vi "Pre-Install Custom Action.vi"(10 "Variant":variant) -> (0 "error out":errorcluster)   [LabVIEW 2021]
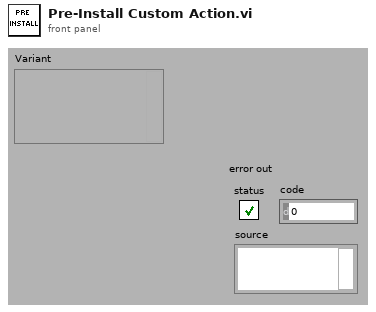
[diagram p1: front panel]
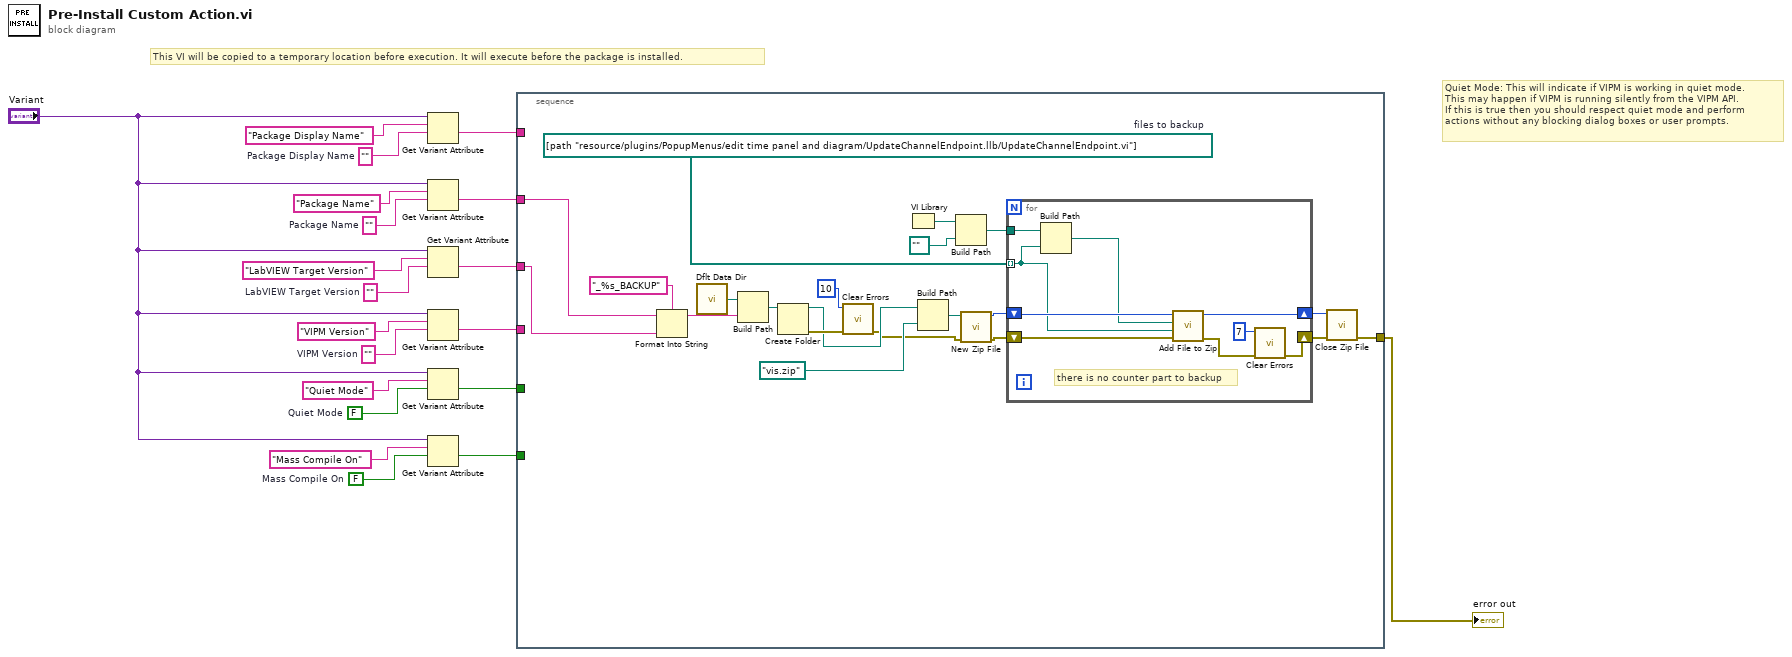
[diagram p0: block diagram]
diagram:
  w2 = FALSE  # Mass Compile On
  w4 = ""  # Package Display Name
  w11 = FALSE  # Quiet Mode
  w14 = ""  # VIPM Version
  w16 = ""  # LabVIEW Target Version
  w18 = ""  # Package Name
  # "Quiet Mode: This will indicate if VIPM is working in quiet mode.\nThis may happen if VIPM is running silently from the VIPM API.\nIf this is true then you should respect quiet mode and perform\nactions without any blocking dialog boxes or user prompts."
  # "This VI will be copied to a temporary location before execution. It will execute before the package is installed."
  n1 = Get Variant Attribute(Variant="Variant", name="Package Display Name", default value (empty Variant)=w4) -> (value=w10:string)  [unwired: 1 in, 3 out]
  n2 = Get Variant Attribute(Variant="Variant", name="Package Name", default value (empty Variant)=w18) -> (value=w9:string)  [unwired: 1 in, 3 out]
  n3 = Get Variant Attribute(Variant="Variant", name="LabVIEW Target Version", default value (empty Variant)=w16) -> (value=w8:string)  [unwired: 1 in, 3 out]
  n4 = Get Variant Attribute(Variant="Variant", name="VIPM Version", default value (empty Variant)=w14) -> (value=w7:string)  [unwired: 1 in, 3 out]
  n5 = Get Variant Attribute(Variant="Variant", name="Quiet Mode", default value (empty Variant)=w11) -> (value=w6:bool)  [unwired: 1 in, 3 out]
  n6 = Get Variant Attribute(Variant="Variant", name="Mass Compile On", default value (empty Variant)=w2) -> (value=w5:bool)  [unwired: 1 in, 3 out]
  n7 = stacked-sequence {
    tunnel: w10 -> [_]
    tunnel: w9 -> [w40]
    tunnel: w8 -> [w39]
    tunnel: w7 -> [_]
    tunnel: w6 -> [_]
    tunnel: w5 -> [_]
    tunnel: [w21] -> w1
    frame #0 {
      w29 = path[] [path "resource/plugins/PopupMenus/edit time panel and diagram/UpdateChannelEndpoint.llb/UpdateChannelEndpoint.vi"]  # files to backup
      n8 = Format Into String(format string="_%s_BACKUP", initial string=w40, w39) -> (resulting string=w27:string)  [unwired: 1 in, 1 out]
      n9 = call <vilib>:"Dflt Data Dir.vi"() -> ("App:Default Data Directory"=w28:path)
      n10 = Build Path(base path=w28, name or relative path=w27) -> (appended path=w26:path)
      n11 = Create Folder(path (use dialog)=w26) -> (created path=w23:path, error out=w25:errorcluster)  [unwired: 2 in, 1 out]
      n12 = call <vilib>:"Clear Errors.vi"("error in (no error)"=w25, "specific error code to clear (0: all)"=10) -> ("error out"=w22:errorcluster)  [unwired: 4 in, 1 out]
      n13 = VI Library() -> (path=w34:path)
      n14 = Build Path(base path=w23, name or relative path=path "vis.zip") -> (appended path=w30:path)
      n15 = Build Path(base path=w34, name or relative path=path "..") -> (appended path=w32:path)
      n16 = call <vilib>:"New Zip File.vi"("error in (no error)"=w22, "target"=w30) -> ("error out"=w37:errorcluster, "zip file out"=w38:i64)  [unwired: 3 in, 1 out]
      n17 = for {
        tunnel: w29 -> [w42] mode=indexing
        shift-right: [w45] -> w36
        shift-left: w37 -> [w47]
        shift-right: [w48] -> w35
        shift-left: w38 -> [w49]
        tunnel: w32 -> [w43]
        # "there is no counter part to backup"
        n18 = Build Path(base path=w43, name or relative path=w42) -> (appended path=w46:path)
        n19 = call <vilib>:"Add File to Zip.vi"("error in (no error)"=w47, "destination path in zip"=w42, "source file path"=w46, "zip file in"=w49) -> ("error out"=w50:errorcluster, "zip file out"=w48:i64)  [unwired: 6 in]
        n20 = call <vilib>:"Clear Errors.vi"("error in (no error)"=w50, "specific error code to clear (0: all)"=7) -> ("error out"=w45:errorcluster)  [unwired: 4 in, 1 out]
      }
      n21 = call <vilib>:"Close Zip File.vi"("error in (no error)"=w36, "zip file in"=w35) -> ("error out"=w21:errorcluster)  [unwired: 5 in]
    }
  }
  "error out" <- w1
